vi "testFileLoading.vi"(9 "Ticks Per Rev":dbl, 10 "Wheel Radius(inches)":dbl, 11 "file path (use dialog)":path) -> ()   [LabVIEW 2014]
panel:
  out "output cluster":T1
  out "World X":dbl[](array[numeric]) format="%.2f"
  out "World Y":dbl[](array[numeric]) format="%.2f"
  out "Y Array":dbl[](array[numeric]) format="%.2f"
  out "X Array":dbl[](array[numeric]) format="%.2f"
  in  "error in":errorcluster
  out "error out":errorcluster
  out "Lines":string[](array[string])
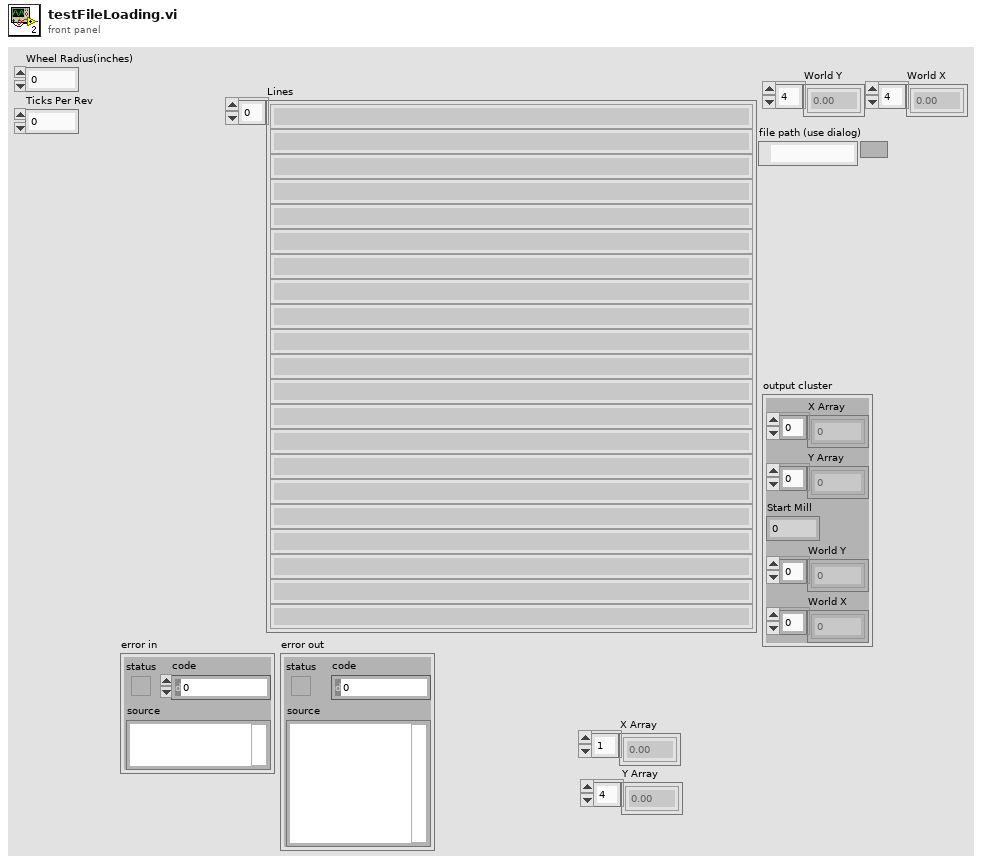
[diagram p1: front panel]
types:
  T1 = cluster{"X Array":dbl[], "Y Array":dbl[], "Start Mill":i32, "World Y":dbl[], "World X":dbl[]}
  T2 = enum16{"open", "replace", "create", "open or create", "replace or create", "replace or create with confirmation"}
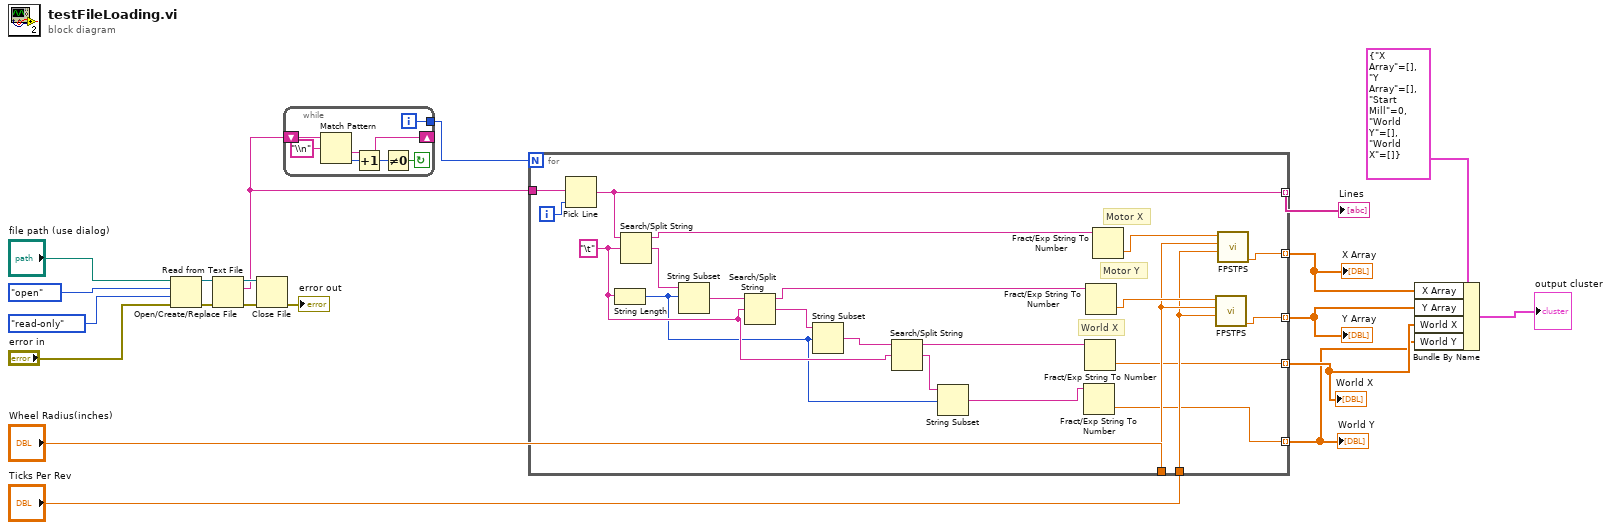
[diagram p0: block diagram]
diagram:
  n1 = Open/Create/Replace File(file path (use dialog)="file path (use dialog)", error in="error in", operation (0:open)=T2."open", access (0:read/write)=enum16{"read/write", "read-only", "write-only"}."read-only") -> (refnum out=w20:refnum<file>, error out=w19:errorcluster)  [unwired: 2 in, 1 out]
  n2 = Read from Text File(file (use dialog)=w20, error in=w19) -> (refnum out=w16:refnum<file>, text=w12:string, error out=w17:errorcluster)  [unwired: 2 in, 1 out]
  n3 = Close File(refnum=w16, error in=w17) -> (error out=→"error out":errorcluster)  [unwired: 1 out]
  n4 = while {
    tunnel: [w21] -> w9
    shift-left: w12 -> [w27]
    shift-right: [w25] -> _
    i -> [w21]
    stop <- w22 continue-if-true
    n5 = Match Pattern(string=w27, regular expression="\\n") -> (after substring=w25:string, offset past match=w24:i32)  [unwired: 1 in, 2 out]
    n6 = Increment(x=w24) -> (x+1=w23:i32)
    n7 = Not Equal To 0?(x=w23) -> (x != 0?=w22:bool)
  }
  n8 = for {
    N: w9 -> [_]
    tunnel: w12 -> [w48]
    tunnel: [w47] -> w15 mode=indexing
    tunnel: [w44] -> w7 mode=indexing
    tunnel: [w42] -> w6 mode=indexing
    tunnel: "Wheel Radius(inches)" -> [w41]
    tunnel: "Ticks Per Rev" -> [w40]
    tunnel: [w29] -> w3 mode=indexing
    tunnel: [w28] -> w2 mode=indexing
    i -> [w49]
    w34 = "\t" ("search string/char (-)")
    # "World X"
    # "Motor Y"
    # "Motor X"
    n9 = Pick Line(multi-line string=w48, line index=w49) -> (output string=w47:string)  [unwired: 1 in]
    n10 = String Length(string=w34) -> (length=w30:i32)
    n11 = Search/Split String(string=w47, search string/char (-)=w34) -> (substring before match=w39:string, match + rest of string=w46:string)  [unwired: 1 in, 1 out]
    n12 = String Subset(string=w46, offset (0)=w30) -> (substring=w38:string)  [unwired: 1 in]
    n13 = Search/Split String(string=w38, search string/char (-)=w34) -> (substring before match=w37:string, match + rest of string=w36:string)  [unwired: 1 in, 1 out]
    n14 = String Subset(string=w36, offset (0)=w30) -> (substring=w35:string)  [unwired: 1 in]
    n15 = Search/Split String(string=w35, search string/char (-)=w34) -> (substring before match=w33:string, match + rest of string=w32:string)  [unwired: 1 in, 1 out]
    n16 = String Subset(string=w32, offset (0)=w30) -> (substring=w31:string)  [unwired: 1 in]
    n17 = Fract/Exp String To Number(string=w31) -> (number=w28:dbl)  [unwired: 3 in, 1 out]
    n18 = Fract/Exp String To Number(string=w33) -> (number=w29:dbl)  [unwired: 3 in, 1 out]
    n19 = Fract/Exp String To Number(string=w37) -> (number=w43:dbl)  [unwired: 3 in, 1 out]
    n20 = Fract/Exp String To Number(string=w39) -> (number=w45:dbl)  [unwired: 3 in, 1 out]
    n21 = call "FPSTPS.vi"("Ticks Per Rev"=w40, "Wheel Radius(inches)"=w41, "Feet Per Second"=w43) -> ("ticks/sec"=w42:dbl)  [unwired: 5 in, 3 out]
    n22 = call "FPSTPS.vi"("Ticks Per Rev"=w40, "Wheel Radius(inches)"=w41, "Feet Per Second"=w45) -> ("ticks/sec"=w44:dbl)  [unwired: 5 in, 3 out]
  }
  "Lines" <- w15
  "X Array" <- w7
  "Y Array" <- w6
  "World Y" <- w2
  "World X" <- w3
  n23 = Bundle By Name(cluster=T1 {"X Array"=[], "Y Array"=[], "Start Mill"=0, "World Y"=[], "World X"=[]} ("input cluster"), "X Array"=w7, "Y Array"=w6, "World X"=w3, "World Y"=w2) -> (→"output cluster":T1)
